vi "Main.vi"() -> ()   [LabVIEW 2018, in "Stream Data.lvlib"]
doc: "This template is based off of the Queued Message Handler design pattern and the Queued Message Handler project template that ships with LabVIEW.\n\nThe main difference is that the queue is private to this module and communication between modules is performed via Broadcast and Request events.\n\nRequest events are wrapped in public API methods and are handled in the Event Handling Loop (EHL) of this VI. Any module can register for Broadcast events sent by this module. The EHL generates messages based on user interface actions.\n\nThe Message Handling Loop (MHL) processes messages generated by the EHL, or by other messages. The messages are string values, so new messages can be added easily to the Message Cases case structure in the MHL. Each message cluster can also provide an optional value for Message Data, which is a variant that can be converted to whatever message-specific data is required.\n_____\nBased on Delacor QMH Project Template 4.2.1.64."
uses:
  Stream Data.lvlib
  <vilib>/Delacor/Delacor QMH/Libraries/Module Admin_class/Delacor_lib_QMH_Module Admin.lvclass
  Private API/Typedefs/CTL_Variable_to_pass.ctl
  Private API/Data.lvclass
  <vilib>/Delacor/Delacor QMH/Libraries/Message Queue_class/Delacor_lib_QMH_Message Queue.lvclass/Delacor_lib_QMH_Message Queue.ctl
  Stop Argument--cluster.ctl
  <vilib>/Delacor/Delacor QMH/Libraries/Module Admin_class/Delacor_lib_QMH_Module Admin.lvclass/Delacor_lib_QMH_Module Admin.ctl
  Send Frame Argument--cluster.ctl
  SubVi's/Controls/CTL_Full_data_frame.ctl
  SubVi's/Controls/CTL_Animal_Coordinates_and_Speed.ctl
  SubVi's/Controls/CTL_Measurements_and_Statistics.ctl
  Open Serial Port Argument--cluster.ctl
  Change Serial Port Argument--cluster.ctl
  Close Serial Port Argument--cluster.ctl
  Update Status Argument--cluster.ctl
  Prepare to Exit Argument--cluster.ctl
  <vilib>/Utility/miscctls.llb/LVPointTypeDef.ctl
  Private API/Data.lvclass/Data.ctl
  <vilib>/Instr/_visa.llb/VISA Open Access Mode.ctl
  <vilib>/Instr/_visa.llb/VISA Set IO Buffer Mask.ctl
  <vilib>/Utility/error.llb/DialogType.ctl
  <vilib>/Delacor/Delacor QMH/Libraries/Message Queue_class/Delacor_lib_QMH_Enqueue Message (Single).vi
  <vilib>/Delacor/Delacor QMH/Libraries/Module Admin_class/Delacor_lib_QMH_Get External Launch.vi
  Private API/Methods/Read Port Opened.vi
  Private API/Methods/Read Serial Port.vi
  Private API/Methods/Write Serial Port.vi
  Private API/Methods/Write Port Opened.vi
  Private API/Methods/Write Status.vi
  <vilib>/Utility/error.llb/Error Cluster From Error Code.vi
  <vilib>/Instr/_visa.llb/VISA Configure Serial Port (Instr).vi
  <vilib>/ErrorRing/Error Ring.xnode
  <vilib>/Delacor/Delacor QMH/Libraries/Message Queue_class/Delacor_lib_QMH_Message Queue.lvclass
  Tracker.lvlib
panel:
  out "Bytes written":u32
  out "Bytes sent":u32
  in  "Line End":u16(ring)=4 items=["Nothing", "Tab", "CR", "LF", "CRLF"]
  in  "Line Start":u16(ring) items=["Nothing", "Tab"]
  in  "Variable 8":T1=enum."Speed, mm/s"
  in  "Variable 7":T1=enum."Zone #"
  in  "Variable 6":T1=enum."Y"
  in  "Variable 5":T1=enum."X"
  in  "Variable 4":T1=enum."alpha"
  in  "Variable 3":T1=enum."phi"
  in  "Variable 2":T1=enum."R"
  in  "Variable 1":T1=enum."timestamp (SW)"
  in  "Mode":bool
  in  "Enable":bool
  in  "Send test frame":bool
  in  "Serial Port":refnum<visa-resource-name>
  in  "Simulate MHL Error":bool
  in  "Simulate EHL Error":bool
  out "error out":errorcluster
  in  "Module Admin":refnum<class "Delacor_lib_QMH_Module Admin.lvclass">
  out "Status":string
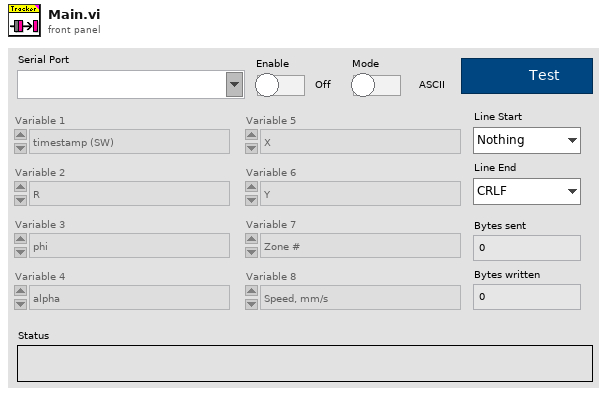
[diagram p1: front panel]
types:
  T1 = typedef "Stream Data.lvlib/CTL_Variable_to_pass.ctl" = enum16{"since ON, ms", "delta time, ms", "timestamp (SW)", "R", "phi", "alpha", "X", "Y", "Zone #", "Run percentage", "Speed, mm/s"}
  T2 = typedef "Stream Data.lvlib/Request Events--cluster.ctl" = cluster{"Stop Module":refnum<user-event>, "Show Panel":refnum<user-event>, "Hide Panel":refnum<user-event>, "Get Module Execution Status":refnum<user-event>, "Show Diagram":refnum<user-event>, "Send Frame":refnum<user-event>, "Open Serial Port":refnum<user-event>, "Change Serial Port":refnum<user-event>, "Close Serial Port":refnum<user-event>, "Update Status":refnum<user-event>, "Prepare to Exit":refnum<user-event>}
  T3 = enum32{"invalid lock state", "Not Locked", "Locked (No Password)", "Password-protected"}
  T4 = typedef "Stream Data.lvlib/Stop Argument--cluster.ctl" = cluster{"Origin":string, "Exit via Stop Module Req?":bool, "Wait for Module to stop?":bool}
  T5 = typedef "Stream Data.lvlib/Send Frame Argument--cluster.ctl" = cluster{"Data in":T6}
  T6 = typedef "Tracker.lvlib/CTL_Full_data_frame.ctl" = cluster{"Times":cluster{"ms since ON":u32, "delta time":u32, "Frame timestamp":timestamp}, "TTLs":cluster{"TTL input":i16, "TTL output":i16}, "Animal coordinates":T7, "Magnets coords raw":cluster{"X1 raw":dbl, "Y1 raw":dbl, "X2 raw":dbl, "Y2 raw":dbl}, "Measurements and statistics":T8}
  T7 = typedef "Tracker.lvlib/CTL_Animal_Coordinates_and_Speed.ctl" = cluster{"R from center":dbl, "phi (mouse angular position in the cage)":dbl, "alpha (mouse rot. angle)":dbl, "X":dbl, "Y":dbl, "theta (from center towards mouse)":dbl, "beta (cage rot. against mouse)":dbl, "w (mouse angle to wall)":dbl, "Speed (filtered)":dbl}
  T8 = typedef "Tracker.lvlib/CTL_Measurements_and_Statistics.ctl" = cluster{"Zone #":i8, "Histogram":dbl[], "Running, perc. of time":dbl, "Run, meters":dbl, "Avg. speed":dbl}
  T9 = typedef "Stream Data.lvlib/Open Serial Port Argument--cluster.ctl" = cluster{"Serial Port":refnum<visa-resource-name>}
  T10 = typedef "Stream Data.lvlib/Change Serial Port Argument--cluster.ctl" = cluster{"Serial Port":refnum<visa-resource-name>}
  T11 = typedef "Stream Data.lvlib/Close Serial Port Argument--cluster.ctl" = cluster{"Serial Port":refnum<visa-resource-name>}
  T12 = typedef "Stream Data.lvlib/Update Status Argument--cluster.ctl" = cluster{"Status":string}
  T13 = typedef "Stream Data.lvlib/Prepare to Exit Argument--cluster.ctl" = cluster{"Boolean":bool}
  T14 = typedef "LVPointTypeDef.ctl" = cluster{"Horizontal":i16, "Vertical":i16}
  T15 = enum32{"Invalid", "Standard", "Closed", "Hidden", "Minimized", "Maximized"}
  T16 = typedef "VISA Set IO Buffer Mask.ctl" = u16
  T17 = typedef "VISA Open Access Mode.ctl" = u32
  T18 = typedef "DialogType.ctl" = u16
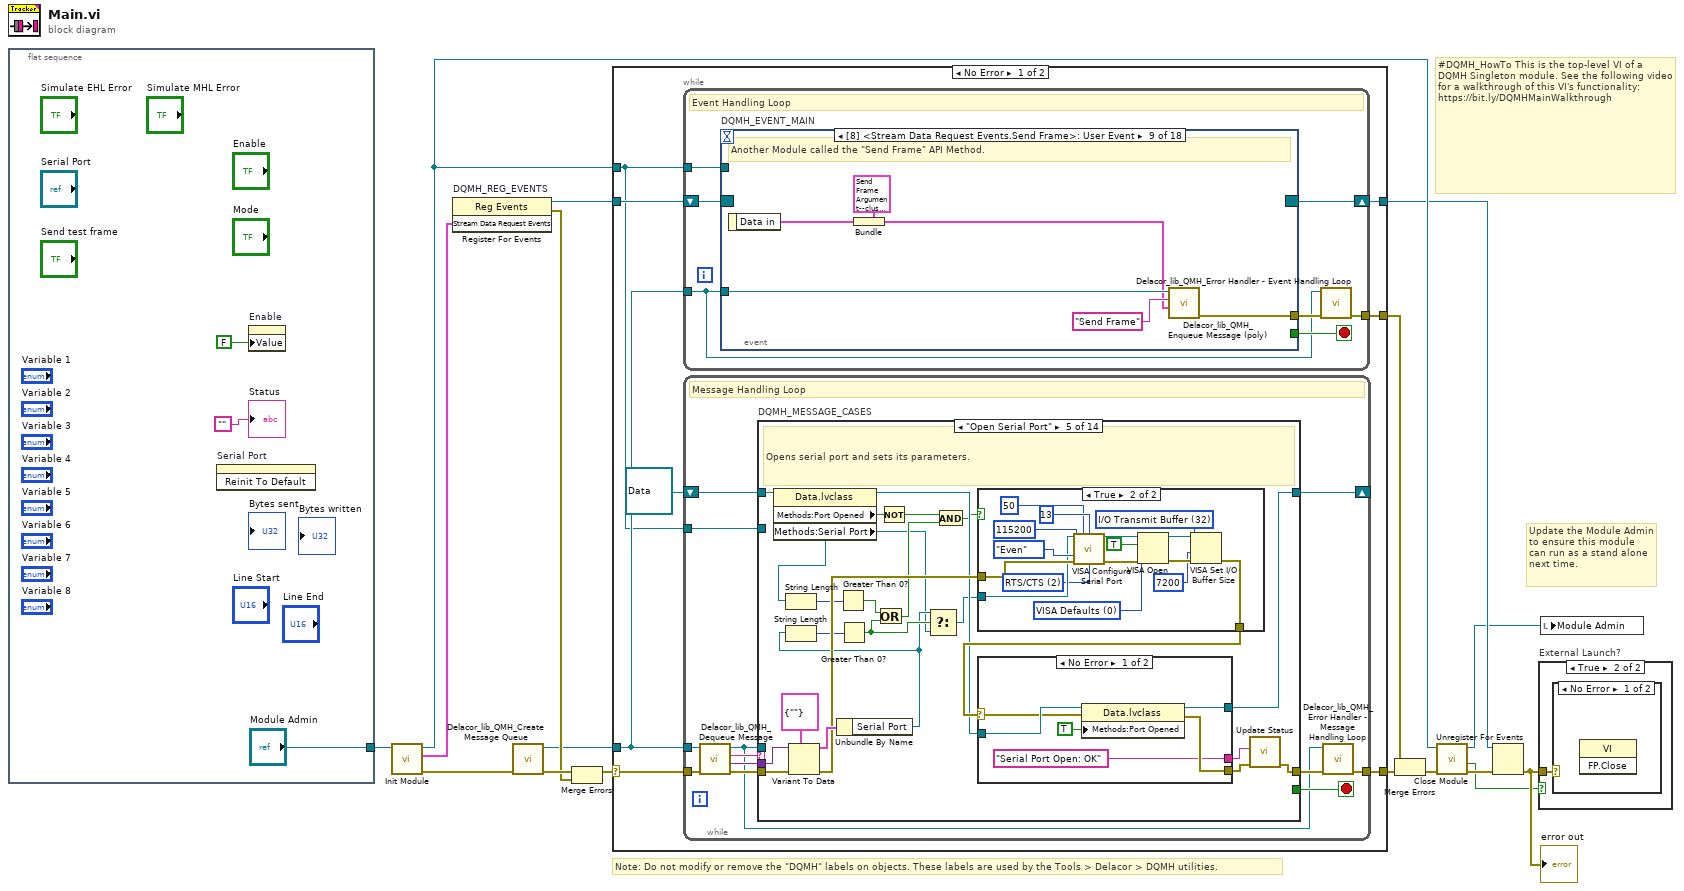
[diagram p0: block diagram]
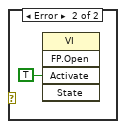
[diagram p3: hidden frame]
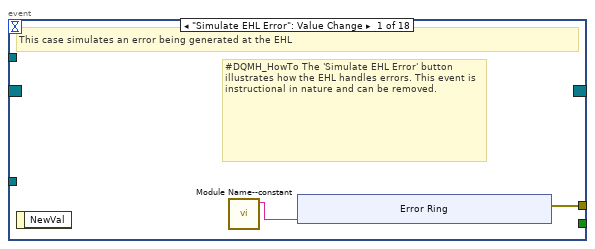
[diagram p4: hidden frame]
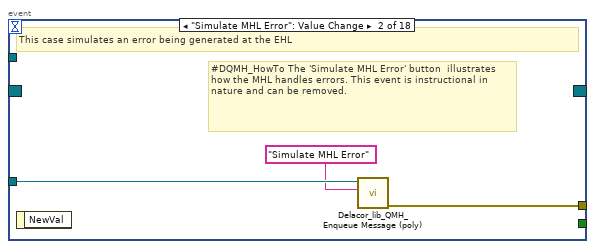
[diagram p5: hidden frame]
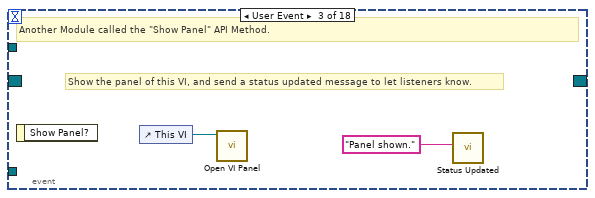
[diagram p6: hidden frame]
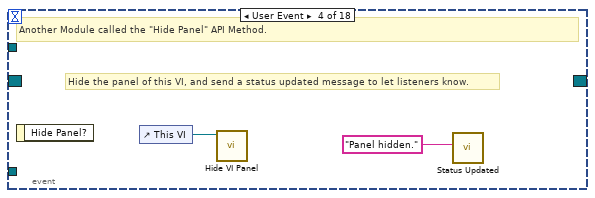
[diagram p7: hidden frame]
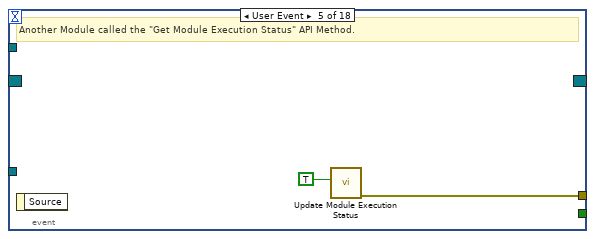
[diagram p8: hidden frame]
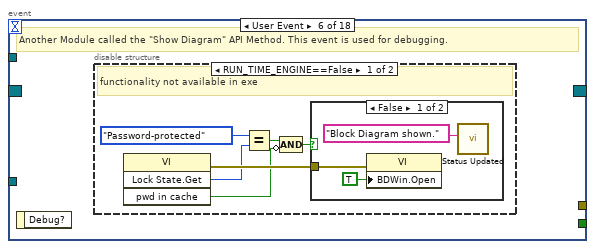
[diagram p9: hidden frame]
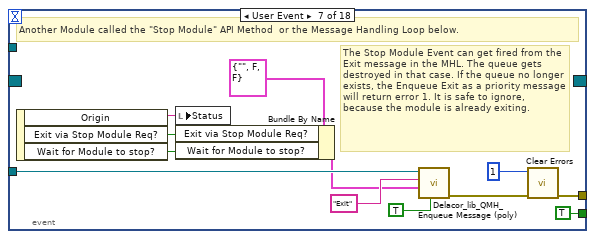
[diagram p12: hidden frame]
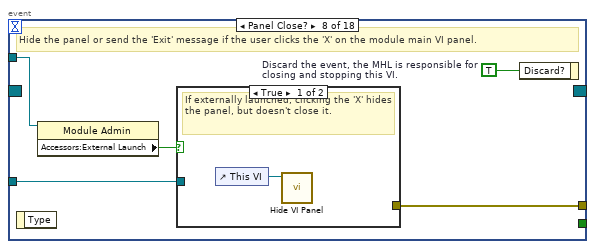
[diagram p13: hidden frame]
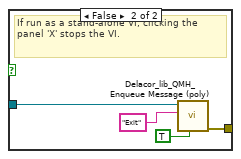
[diagram p14: hidden frame]
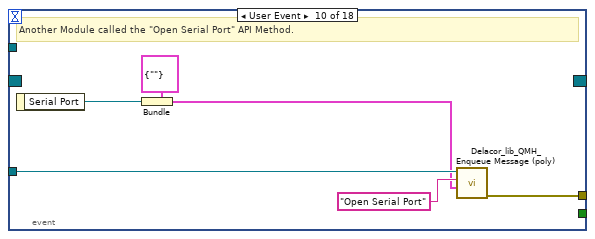
[diagram p15: hidden frame]
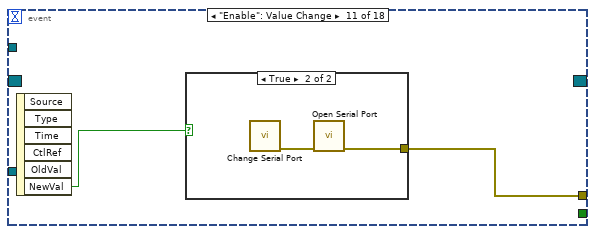
[diagram p16: hidden frame]
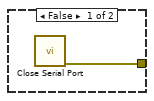
[diagram p17: hidden frame]
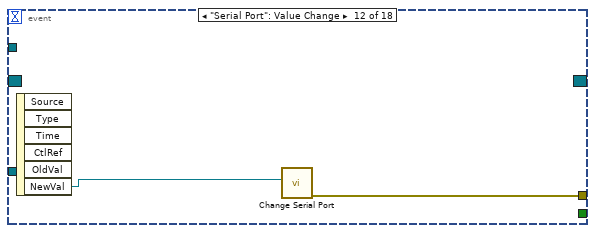
[diagram p18: hidden frame]
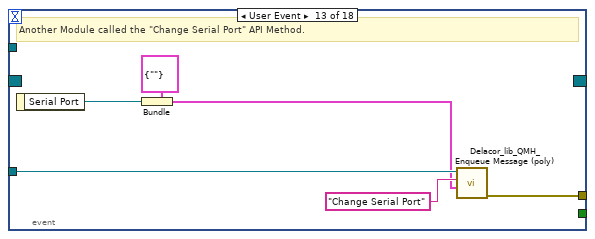
[diagram p19: hidden frame]
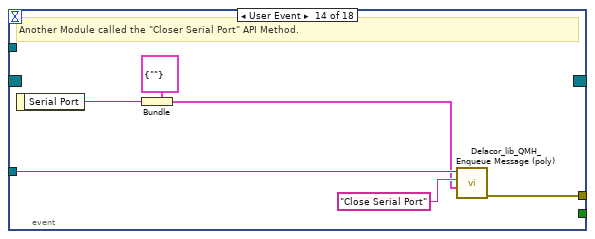
[diagram p20: hidden frame]
diagram:
  # "#DQMH_HowTo This is the top-level VI of a DQMH Singleton module. See the following video for a walkthrough of this VI's functionality: https://bit.ly/DQMHMainWalkthrough"
  # "Note: Do not modify or remove the \"DQMH\" labels on objects. These labels are used by the Tools > Delacor > DQMH utilities."
  # "Update the Module Admin to ensure this module can run as a stand alone next time."
  n1 = flat-sequence {
    tunnel: ["Module Admin"] -> w1
    frame #0 {
      n2 = invoke on="Serial Port" class="VISAName" method="Reinit To Default"() -> ()  [unwired: 3 in, 3 out]
      n3 = property on="Enable" class="Bool (strict)"("Value"=FALSE ("Enable")) -> ()  [unwired: 2 in, 2 out]
      "Status" <- ""
    }
  }
  n4 = call "Init Module.vi"("Singleton Module Admin in"=w1) -> ("error out"=w16:errorcluster, "Stream Data Request Events"=w5:T2, "Singleton Module Admin out"=w8:refnum<class "Delacor_lib_QMH_Module Admin.lvclass">)  [unwired: 8 in]
  n5 = register-events "DQMH_REG_EVENTS"(w5) -> (reference out=w6:refnum<event-registration>, error out=w9:errorcluster)  [unwired: 2 in]
  n6 = call <vilib>:"Delacor_lib_QMH_Create Message Queue.vi"("error in (no error)"=w16) -> ("error out"=w11:errorcluster, "Message Queue"=w4:refnum<class "Delacor_lib_QMH_Message Queue.lvclass">)  [unwired: 9 in]
  n7 = Merge Errors(w11, w9) -> (w10:errorcluster)
  n8 = case shown="No Error" w10 {
    selector: w10 -> [w26 w379]
    tunnel: [w28 w379] -> w17
    tunnel: [w25 w376] -> w7
    tunnel: w6 -> [w24 w376]
    tunnel: w4 -> [w23 _]
    tunnel: [w27 _] -> w14
    tunnel: w8 -> [w22 w372]
    frame No Error {
      n9 = while {
        tunnel: w23 -> [w29]
        shift-right: [w32] -> w25
        shift-left: w24 -> [w33]
        tunnel: [w34] -> w27
        tunnel: w22 -> [w30]
        stop <- w31 stop-if-true
        # "Event Handling Loop"
        n10 = event "DQMH_EVENT_MAIN" shown="[8] <Stream Data Request Events.Send Frame>: User Event" {
          selector: w33 -> [_ _ _ _ _ _ _ _ _ _ _ _ _ _ _ _ _ _]
          dyn-events: [_ _ _ _ _ _ _ _ _ _ _ _ _ _ _ _ _ _] -> w32
          timeout: _ -> [_ _ _ _ _ _ _ _ _ _ _ _ _ _ _ _ _ _]
          tunnel: [_ _ _ _ _ _ TRUE ("Discard?") _ _ _ _ _ _ _ _ _ _ _] -> w31
          tunnel: w29 -> [_ w46 _ _ _ _ w70 w77 w90 w96 _ _ w109 w115 w121 _ _ w131]
          tunnel: [w37 w47 _ _ w53 _ w73 w79 w85 w91 w97 w102 w104 w110 w116 w123 _ w126] -> w35
          tunnel: w30 -> [_ _ _ _ _ _ _ w76 _ _ _ _ _ _ _ _ _ _]
          event "Simulate EHL Error": Value Change {
            # "#DQMH_HowTo The 'Simulate EHL Error' button  illustrates how the EHL handles errors. This event is instructional in nature and can be removed."
            # "This case simulates an error being generated at the EHL"
            n11 = event-data() -> ()  [unwired: 1 in, 1 out]
            n12 = call "Module Name--constant.vi"() -> ("Module Name"=w36:string)  [unwired: 11 in]
            n13 = xnode "Error Ring"("parameter 0"=w36) -> ("error out"=w37:errorcluster)
          }
          event "Simulate MHL Error": Value Change {
            # "#DQMH_HowTo The 'Simulate MHL Error' button  illustrates how the MHL handles errors. This event is instructional in nature and can be removed."
            # "This case simulates an error being generated at the EHL"
            n14 = event-data() -> ()  [unwired: 1 in, 1 out]
            n15 = call-poly <vilib>:"Delacor_lib_QMH_Enqueue Message (poly).vi"("Message"="Simulate MHL Error", "Message Queue in"=w46) -> ("error out"=w47:errorcluster)  [unwired: 8 in, 1 out]
          }
          event User Event {
            # "Show the panel of this VI, and send a status updated message to let listeners know."
            # "Another Module called the \"Show Panel\" API Method."
            n16 = event-data() -> ()  [unwired: 1 in, 1 out]
            n17 = control-ref of="This VI"() -> (w49:refnum<vi>)
            n18 = call "Open VI Panel.vi"("VI"=w49) -> ()  [unwired: 10 in, 1 out]
            n19 = call "Status Updated.vi"("Status"="Panel shown." ("format string")) -> ()  [unwired: 10 in, 1 out]
          }
          event User Event {
            # "Hide the panel of this VI, and send a status updated message to let listeners know."
            # "Another Module called the \"Hide Panel\" API Method."
            n20 = event-data() -> ()  [unwired: 1 in, 1 out]
            n21 = control-ref of="This VI"() -> (w51:refnum<vi>)
            n22 = call "Hide VI Panel.vi"("VI"=w51) -> ()  [unwired: 10 in, 1 out]
            n23 = call "Status Updated.vi"("Status"="Panel hidden." ("format string")) -> ()  [unwired: 10 in, 1 out]
          }
          event User Event {
            # "Another Module called the \"Get Module Execution Status\" API Method."
            n24 = event-data() -> ()  [unwired: 1 in, 1 out]
            n25 = call "Update Module Execution Status.vi"("Running?"=TRUE) -> ("error out"=w53:errorcluster)  [unwired: 10 in]
          }
          event User Event {
            # "Another Module called the \"Show Diagram\" API Method. This event is used for debugging."
            n26 = event-data() -> ()  [unwired: 1 in, 1 out]
            n27 = disable-structure shown="RUN_TIME_ENGINE==False" {
              frame condition #0 (active) {
                # "functionality not available in exe"
                n28 = invoke class="VI" method="Lock State.Get"() -> (error out=w59:errorcluster, "Get Lock State"=w58:T3, "pwd in cache"=w55:bool)  [unwired: 4 in, 1 out]
                n29 = Equal?(x=T3."Password-protected", y=w58) -> (x = y?=w56:bool)
                n30 = Compound Arithmetic op=AND(w56, invert w55) -> (w54:bool)
                n31 = case shown="False" w54 {
                  tunnel: w59 -> [w62 _]
                  frame False {
                    n32 = property class="VI"(error in=w62, "BDWin.Open"=TRUE ("Block Diagram Window:Open")) -> ()  [unwired: 1 in, 2 out]
                    n33 = call "Status Updated.vi"("Status"="Block Diagram shown." ("format string")) -> ()  [unwired: 10 in, 1 out]
                  }
                  frame True {
                    # "Password-protected VI, and the password is not in the cache. Do not show the diagram."
                  }
                }
              }
              frame condition #1 {
              }
            }
          }
          event User Event {
            # "The Stop Module Event can get fired from the Exit message in the MHL. The queue gets destroyed in that case. If the queue no longer exists, the Enqueue Exit as a priority message will return error 1. It is safe to ignore, because the module is already exiting."
            # "Another Module called the \"Stop Module\" API Method  or the Message Handling Loop below."
            n34 = event-data() -> ("Origin"=w69:string, "Exit via Stop Module Req?"=w65:bool, "Wait for Module to stop?"=w64:bool)  [unwired: 1 in]
            n35 = local write "Status"(w69) -> ()
            n36 = Bundle By Name(cluster=T4 {"Origin"="", "Exit via Stop Module Req?"=FALSE, "Wait for Module to stop?"=FALSE} ("Stop Argument"), "Exit via Stop Module Req?"=w65, "Wait for Module to stop?"=w64) -> (w63:T4)
            n37 = call-poly <vilib>:"Delacor_lib_QMH_Enqueue Message (poly).vi"("Priority Message? (F)"=TRUE, "Message Data"=w63, "Message"="Exit", "Message Queue in"=w70) -> ("error out"=w74:errorcluster)  [unwired: 6 in, 1 out]
            n38 = call <vilib>:"Clear Errors.vi"("error in (no error)"=w74, "specific error code to clear (0: all)"=1) -> ("error out"=w73:errorcluster)  [unwired: 4 in, 1 out]
          }
          event Panel Close? {
            w78 = TRUE  # Discard the event, the MHL is responsible for closing and stopping this VI.
            # "Hide the panel or send the 'Exit' message if the user clicks the 'X' on the module main VI panel."
            n39 = event-data() -> ()  [unwired: 1 in, 1 out]
            n40 = property class="Module Admin"(reference=w76) -> ("Accessors:External Launch"=w75:bool)  [unwired: 1 in, 2 out]
            n41 = case shown="True" w75 {
              tunnel: w77 -> [_ w83]
              tunnel: [_ w84] -> w79
              frame True {
                # "If externally launched, clicking the 'X' hides the panel, but doesn't close it."
                n42 = control-ref of="This VI"() -> (w80:refnum<vi>)
                n43 = call "Hide VI Panel.vi"("VI"=w80) -> ()  [unwired: 10 in, 1 out]
              }
              frame False {
                # "If run as a stand-alone VI, clicking the panel 'X' stops the VI."
                n44 = call-poly <vilib>:"Delacor_lib_QMH_Enqueue Message (poly).vi"("Priority Message? (F)"=TRUE, "Message"="Exit", "Message Queue in"=w83) -> ("error out"=w84:errorcluster)  [unwired: 7 in, 1 out]
              }
            }
            n45 = event-data("Discard?"=w78) -> ()  [unwired: 1 in, 1 out]
          }
          event User Event {
            # "Another Module called the \"Send Frame\" API Method."
            n46 = event-data() -> ("Data in"=w86:T6)  [unwired: 1 in]
            n47 = Bundle(cluster=T5 {"Data in"={"Times"={"ms since ON"=0, "delta time"=0, "Frame timestamp"=timestamp(0 s since 1904-01-01)}, "TTLs"={"TTL input"=0, "TTL output"=0}, "Animal coordinates"={"R from center"=0.0, "phi (mouse angular position in the cage)"=0.0, "alpha (mouse rot. angle)"=0.0, "X"=0.0, "Y"=0.0, "theta (from center towards mouse)"=0.0, "beta (cage rot. against mouse)"=0.0, "w (mouse angle to wall)"=0.0, "Speed (filtered)"=0.0}, "Magnets coords raw"={"X1 raw"=0.0, "Y1 raw"=0.0, "X2 raw"=0.0, "Y2 raw"=0.0}, "Measurements and statistics"={"Zone #"=0, "Histogram"=[], "Running, perc. of time"=0.0, "Run, meters"=0.0, "Avg. speed"=0.0}}} ("Send Frame Argument"), "Data in"=w86) -> (w87:T5)
            n48 = call-poly <vilib>:"Delacor_lib_QMH_Enqueue Message (poly).vi"("Message Data"=w87, "Message"="Send Frame", "Message Queue in"=w90) -> ("error out"=w85:errorcluster)  [unwired: 7 in, 1 out]
          }
          event User Event {
            # "Another Module called the \"Open Serial Port\" API Method."
            n49 = event-data() -> ("Serial Port"=w92:refnum<visa-resource-name>)  [unwired: 1 in]
            n50 = Bundle(cluster=T9 {"Serial Port"=""} ("Open Serial Port Argument"), "Serial Port"=w92) -> (w93:T9)
            n51 = call-poly <vilib>:"Delacor_lib_QMH_Enqueue Message (poly).vi"("Message Data"=w93, "Message"="Open Serial Port", "Message Queue in"=w96) -> ("error out"=w91:errorcluster)  [unwired: 7 in, 1 out]
          }
          event "Enable": Value Change {
            n52 = event-data() -> ("NewVal"=w98:bool)  [unwired: 1 in, 5 out]
            n53 = case shown="True" w98 {
              tunnel: [w99 w101] -> w97
              frame False {
                n54 = call "Close Serial Port.vi"() -> ("error out"=w99:errorcluster)  [unwired: 11 in]
              }
              frame True {
                n55 = call "Change Serial Port.vi"() -> ("error out"=w100:errorcluster)  [unwired: 11 in]
                n56 = call "Open Serial Port.vi"("error in (no error)"=w100) -> ("error out"=w101:errorcluster)  [unwired: 10 in]
              }
            }
          }
          event "Serial Port": Value Change {
            n57 = event-data() -> ("NewVal"=w103:refnum<visa-resource-name>)  [unwired: 1 in, 5 out]
            n58 = call "Change Serial Port.vi"("Serial Port"=w103) -> ("error out"=w102:errorcluster)  [unwired: 10 in]
          }
          event User Event {
            # "Another Module called the \"Change Serial Port\" API Method."
            n59 = event-data() -> ("Serial Port"=w105:refnum<visa-resource-name>)  [unwired: 1 in]
            n60 = Bundle(cluster=T10 {"Serial Port"=""} ("Change Serial Port Argument"), "Serial Port"=w105) -> (w106:T10)
            n61 = call-poly <vilib>:"Delacor_lib_QMH_Enqueue Message (poly).vi"("Message Data"=w106, "Message"="Change Serial Port", "Message Queue in"=w109) -> ("error out"=w104:errorcluster)  [unwired: 7 in, 1 out]
          }
          event User Event {
            # "Another Module called the \"Closer Serial Port\" API Method."
            n62 = event-data() -> ("Serial Port"=w111:refnum<visa-resource-name>)  [unwired: 1 in]
            n63 = Bundle(cluster=T11 {"Serial Port"=""} ("Closer Serial Port Argument"), "Serial Port"=w111) -> (w112:T11)
            n64 = call-poly <vilib>:"Delacor_lib_QMH_Enqueue Message (poly).vi"("Message Data"=w112, "Message"="Close Serial Port", "Message Queue in"=w115) -> ("error out"=w110:errorcluster)  [unwired: 7 in, 1 out]
          }
          event User Event {
            # "Another Module called the \"Update Status\" API Method."
            n65 = event-data() -> ("Status"=w117:string)  [unwired: 1 in]
            n66 = Bundle(cluster=T12 {"Status"=""} ("Update Status Argument"), "Status"=w117) -> (w118:T12)
            n67 = call-poly <vilib>:"Delacor_lib_QMH_Enqueue Message (poly).vi"("Message Data"=w118, "Message"="Update Status", "Message Queue in"=w121) -> ("error out"=w116:errorcluster)  [unwired: 7 in, 1 out]
          }
          event "Send test frame": Value Change {
            n68 = event-data() -> ("OldVal"=w125:bool)  [unwired: 1 in, 5 out]
            n69 = property on="Send test frame" class="Bool (strict)"("Value"=w125) -> ()  [unwired: 2 in, 2 out]
            n70 = call "SD_Gen_Random_Frame.vi"() -> ("error out"=w124:errorcluster, "Generated data"=w122:T6)  [unwired: 10 in]
            n71 = call "Send Frame.vi"("error in (no error)"=w124, "Data in"=w122) -> ("error out"=w123:errorcluster)  [unwired: 9 in]
          }
          event Value Change {
            n72 = event-data() -> ()  [unwired: 1 in, 6 out]
          }
          event User Event {
            # "Another Module called the \"Prepare to Exit\" API Method."
            n73 = event-data() -> ("Boolean"=w127:bool)  [unwired: 1 in]
            n74 = Bundle(cluster=T13 {"Boolean"=FALSE} ("Prepare to Exit Argument"), "Boolean"=w127) -> (w128:T13)
            n75 = call-poly <vilib>:"Delacor_lib_QMH_Enqueue Message (poly).vi"("Message Data"=w128, "Message"="Prepare to Exit", "Message Queue in"=w131) -> ("error out"=w126:errorcluster)  [unwired: 7 in, 1 out]
          }
        }
        n76 = call-dynamic "Delacor_lib_QMH_Error Handler - Event Handling Loop.vi"("error in (no error)"=w35, "Message Queue in"=w29) -> ("dup error in"=w34:errorcluster)  [unwired: 8 in, 1 out]
      }
      n77 = while {
        tunnel: w23 -> [w134]
        shift-right: [w138] -> _
        shift-left: refnum<class "Data.lvclass"> refnum ("Stream Data.lvlib:Data.lvclass") -> [w139]
        tunnel: w26 -> [w142]
        tunnel: [w140] -> w28
        tunnel: w22 -> [w132]
        stop <- w137 stop-if-true
        # "Message Handling Loop"
        n78 = call-dynamic "Delacor_lib_QMH_Dequeue Message.vi"("error in (no error)"=w142, "Message Queue in"=w134) -> ("error out"=w141:errorcluster, "Message Data"=w135:variant, "Message"=w136:string, "Message Queue out"=w133:refnum<class "Delacor_lib_QMH_Message Queue.lvclass">)  [unwired: 6 in]
        n79 = case "DQMH_MESSAGE_CASES" shown="\"Open Serial Port\"" w136 {
          selector: w136 -> [_ _ _ _ _ _ _ _ _ _ _ _ _ w359]
          tunnel: w133 -> [_ _ _ _ _ _ _ _ _ _ _ w325 w351 _]
          tunnel: w141 -> [w160 w164 w173 w201 w224 w268 w295 w305 w308 w310 w315 w332 w357 w361]
          tunnel: [w158 w164 w166 w189 w203 w255 w293 w300 w307 w310 w314 w328 w354 w362] -> w143
          tunnel: w139 -> [w145 w163 w170 w200 w223 w267 w294 w304 w306 w309 w312 w327 w350 w360]
          tunnel: [w145 w163 w170 w196 w215 w257 w289 w304 w306 w309 w312 w327 w350 w360] -> w138
          tunnel: [_ _ _ _ _ _ _ _ _ _ _ _ w349 _] -> w137
          tunnel: w135 -> [_ _ w172 w199 w222 w266 w292 w303 _ _ _ w326 w348 _]
          tunnel: w132 -> [w150 _ _ _ _ _ _ _ _ _ _ w324 w343 _]
          frame "Initialize" {
            # "Initialize - Any operation that needs to be done before the module can receive messages. Synchronize Caller Events.vi will inform Start Module.vi that the module has launched and is ready to receive messages. Module Did Init.vi will broadcast that the module initialized."
            n80 = call "Synchronize Caller Events.vi"("error in (no error)"=w160, "Singleton Module Admin in"=w150) -> ("error out"=w159:errorcluster, "Singleton Module Admin out"=w147:refnum<class "Delacor_lib_QMH_Module Admin.lvclass">)  [unwired: 8 in]
            n81 = property class="Module Admin"(reference=w147) -> ("Accessors:External Launch"=w154:bool)  [unwired: 1 in, 2 out]
            n82 = Select(t=T15."Hidden" ("State"), s=w154, f=T15."Standard" ("State")) -> (s? t:f=w151:T15)
            n83 = call "Module Name--constant.vi"() -> ("Module Name"=w157:string)  [unwired: 11 in]
            n84 = property class="VI"("Front Panel.Title"=w157) -> (reference out=w156:refnum<vi>, error out=w162:errorcluster)  [unwired: 2 in]
            n85 = call "Update Status.vi"("Status"="Initial Message" ("Initial Message")) -> ()  [unwired: 10 in, 1 out]
            n86 = call "Module Name--constant.vi"() -> ("Module Name"=w148:string)  [unwired: 11 in]
            n87 = invoke class="VI" method="FP.Open"(reference=w156, error in=w162, "State"=w151) -> (reference out=w155:refnum<vi>, error out=w161:errorcluster)  [unwired: 2 in, 3 out]
            n88 = call "Module Did Init.vi"("error in (no error)"=w159, "Initialized?"=TRUE, "Origin"=w148) -> ("error out"=w158:errorcluster)  [unwired: 8 in]
            n89 = invoke class="VI" method="FP.Center"(reference=w155, error in=w161) -> ()  [unwired: 1 in, 3 out]
            n90 = property on="Pane" class="Pane"("Origin"=T14 {"Horizontal"=0, "Vertical"=0}) -> ()  [unwired: 2 in, 2 out]
          }
          frame "--- Module Specific ---" {
            # "Separator -- The following cases handle messages specific to this Module."
          }
          frame "Send Frame" {
            # "Requests to send a single data frame."
            n91 = property class="Data.lvclass"(reference=w170) -> ("Methods:Port Opened"=w169:bool, "Methods:Serial Port"=w165:refnum<visa-resource-name>)  [unwired: 1 in, 2 out]
            n92 = Variant To Data(error in=w173, type=T5 {"Data in"={"Times"={"ms since ON"=0, "delta time"=0, "Frame timestamp"=timestamp(0 s since 1904-01-01)}, "TTLs"={"TTL input"=0, "TTL output"=0}, "Animal coordinates"={"R from center"=0.0, "phi (mouse angular position in the cage)"=0.0, "alpha (mouse rot. angle)"=0.0, "X"=0.0, "Y"=0.0, "theta (from center towards mouse)"=0.0, "beta (cage rot. against mouse)"=0.0, "w (mouse angle to wall)"=0.0, "Speed (filtered)"=0.0}, "Magnets coords raw"={"X1 raw"=0.0, "Y1 raw"=0.0, "X2 raw"=0.0, "Y2 raw"=0.0}, "Measurements and statistics"={"Zone #"=0, "Histogram"=[], "Running, perc. of time"=0.0, "Run, meters"=0.0, "Avg. speed"=0.0}}} ("Send Frame Argument"), Variant=w172) -> (data=w167:T5, error out=w168:errorcluster)
            n93 = case shown="True" w169 {
              tunnel: w168 -> [w174 w184]
              tunnel: w167 -> [_ w183]
              tunnel: [w174 w181] -> w166
              tunnel: w165 -> [_ w180]
              frame False {
              }
              frame True {
                n94 = local read "Line Start"() -> (w178:u16)
                n95 = local read "Mode"() -> (w185:bool)
                n96 = local read "Line End"() -> (w177:u16)
                n97 = call "SD_Construct_data_string.vi"("Line End"=w177, "Line Start"=w178, "error in (no error)"=w184, "Mode"=w185, "Send Frame Argument"=w183) -> ("error out"=w182:errorcluster, "Total bytes"=w176:i32, "Data string"=w179:string)  [unwired: 4 in]
                n98 = local write "Bytes sent"(w176) -> ()
                n99 = VISA Write(VISA resource name=w180, write buffer=w179, error in (no error)=w182) -> (return count=w175:u32, error out=w181:errorcluster)  [unwired: 1 out]
                n100 = local write "Bytes written"(w175) -> ()
              }
            }
          }
          frame "Change Serial Port" {
            # "Changes current serial port information in the class data."
            n101 = Variant To Data(error in=w201, type=T10 {"Serial Port"=""} ("Change Serial Port Argument"), Variant=w199) -> (data=w197:T10, error out=w195:errorcluster)
            n102 = Unbundle By Name(w197) -> ("Serial Port"=w191:refnum<visa-resource-name>)
            n103 = String Length(string=w191) -> (length=w194:i32)
            n104 = local read "Serial Port"() -> (w192:refnum<visa-resource-name>)
            n105 = Greater Than 0?(x=w194) -> (x > 0?=w193:bool)
            n106 = Select(t=w191, s=w193, f=w192) -> (s? t:f=w186:refnum<visa-resource-name>)
            n107 = property class="Data.lvclass"(reference=w200, error in=w195, "Methods:Serial Port"=w186) -> (reference out=w196:refnum<class "Data.lvclass">, error out=w190:errorcluster)
            n108 = Concatenate Strings("Serial port class data changed to: " ("Status"), w186) -> (w187:string)
            n109 = call "Update Status.vi"("error in (no error)"=w190, "Status"=w187) -> ("error out"=w189:errorcluster)  [unwired: 9 in]
          }
          frame "Open Serial Port" {
            # "Opens serial port and sets its parameters."
            n110 = property class="Data.lvclass"(reference=w223) -> (reference out=w216:refnum<class "Data.lvclass">, "Methods:Port Opened"=w219:bool, "Methods:Serial Port"=w206:refnum<visa-resource-name>)  [unwired: 1 in, 1 out]
            n111 = String Length(string=w206) -> (length=w212:i32)
            n112 = Variant To Data(error in=w224, type=T9 {"Serial Port"=""} ("Open Serial Port Argument"), Variant=w222) -> (data=w220:T9, error out=w218:errorcluster)
            n113 = Unbundle By Name(w220) -> ("Serial Port"=w207:refnum<visa-resource-name>)
            n114 = String Length(string=w207) -> (length=w211:i32)
            n115 = Greater Than 0?(x=w212) -> (x > 0?=w210:bool)
            n116 = Greater Than 0?(x=w211) -> (x > 0?=w208:bool)
            n117 = Or(x=w210, y=w208) -> (x .or. y?=w209:bool)
            n118 = Not(x=w219) -> (.not. x?=w213:bool)
            n119 = Select(t=w207, s=w208, f=w206) -> (s? t:f=w205:refnum<visa-resource-name>)
            n120 = And(x=w213, y=w209) -> (x .and. y?=w214:bool)
            n121 = case shown="True" w214 {
              tunnel: w218 -> [w237 w253]
              tunnel: [w237 w245] -> w217
              tunnel: w205 -> [_ w241]
              frame False {
              }
              frame True {
                w239 = u16 2 items=["None", "XON/XOFF", "RTS/CTS", "XON/XOFF & RTS/CTS", "DTR/DSR", "XON/XOFF & DTR/DSR"] ("flow control (0:none)")
                w243 = T16 32 items=["I/O Receive Buffer"=16, "I/O Transmit Buffer"=32, "I/O Receive and Transmit Buffer"=48] ("Mask")
                w247 = T17 0 items=["VISA Defaults"=0, "Exclusive Lock"=1, "Load Configured Settings"=4] ("Access Mode")
                n122 = call-poly "VISA Configure Serial Port"("VISA resource name"=w241, "timeout (10sec)"=u32 50, "termination char\n(0xA = '\\n' = LF)"=u8 13 ("termination char\n(0xA = '\\n' = LF)"), "baud rate (9600)"=u32 115200, "parity (0:none)"=enum16{"None", "Odd", "Even", "Mark", "Space"}."Even", "error in (no error)"=w253, "flow control (0:none)"=w239) -> ("VISA resource name out"=w249:refnum<visa-resource-name>, "error out"=w248:errorcluster)  [unwired: 7 in]
                n123 = VISA Open(duplicate session (F)=TRUE, access mode=w247, error in (no error)=w248, VISA resource name=w249) -> (VISA resource name=w244:refnum<visa-resource-name>, error out=w246:errorcluster)  [unwired: 1 in]
                n124 = VISA Set I/O Buffer Size(VISA resource name=w244, mask (16)=w243, size (4096)=u32 7200, error in (no error)=w246) -> (error out=w245:errorcluster)  [unwired: 1 out]
              }
            }
            n125 = case shown="No Error" w217 {
              selector: w217 -> [w229 w235]
              tunnel: w216 -> [w230 w236]
              tunnel: [w228 w234] -> w215
              tunnel: [w227 w233] -> w204
              tunnel: ["Serial Port Open: OK" ("Status") "Serial Port Open: FAILED" ("Status")] -> w202
              frame No Error {
                n126 = property class="Data.lvclass"(reference=w230, error in=w229, "Methods:Port Opened"=TRUE ("Port Opened")) -> (reference out=w228:refnum<class "Data.lvclass">, error out=w227:errorcluster)
              }
              frame Error {
                n127 = property class="Data.lvclass"(reference=w236, error in=w235, "Methods:Port Opened"=FALSE ("Port Opened")) -> (reference out=w234:refnum<class "Data.lvclass">, error out=w233:errorcluster)
              }
            }
            n128 = call "Update Status.vi"("error in (no error)"=w204, "Status"=w202) -> ("error out"=w203:errorcluster)  [unwired: 9 in]
          }
          frame "Close Serial Port" {
            # "Closes the previously opened serial port."
            n129 = property class="Data.lvclass"(reference=w267) -> (reference out=w258:refnum<class "Data.lvclass">, "Methods:Port Opened"=w263:bool, "Methods:Serial Port"=w262:refnum<visa-resource-name>)  [unwired: 1 in, 1 out]
            n130 = Variant To Data(error in=w268, type=T11 {"Serial Port"=""} ("Closer Serial Port Argument"), Variant=w266) -> (data=w264:T11, error out=w260:errorcluster)
            n131 = Unbundle By Name(w264) -> ("Serial Port"=w261:refnum<visa-resource-name>)
            n132 = case shown="True" w263 {
              tunnel: w261 -> [_ w279]
              tunnel: w262 -> [_ w285]
              tunnel: w260 -> [w278 w281]
              tunnel: [w278 w280] -> w259
              frame False {
              }
              frame True {
                n133 = String Length(string=w279) -> (length=w287:i32)
                n134 = Greater Than 0?(x=w287) -> (x > 0?=w286:bool)
                n135 = Select(t=w279, s=w286, f=w285) -> (s? t:f=w284:refnum<visa-resource-name>)
                n136 = VISA Flush I/O Buffer(VISA resource name=w284, error in (no error)=w281) -> (VISA resource name out=w283:refnum<visa-resource-name>, error out=w282:errorcluster)  [unwired: 1 in]
                n137 = VISA Close(VISA resource name=w283, error in (no error)=w282) -> (error out=w280:errorcluster)
              }
            }
            n138 = case shown="No Error" w259 {
              selector: w259 -> [w273 w276]
              tunnel: w258 -> [w274 w277]
              tunnel: [w272 w277] -> w257
              tunnel: [w271 w276] -> w256
              tunnel: ["Serial Port Close: OK" ("Status") "Serial Port Close: FAILED" ("Status")] -> w254
              frame No Error {
                n139 = property class="Data.lvclass"(reference=w274, error in=w273, "Methods:Port Opened"=FALSE ("Port Opened")) -> (reference out=w272:refnum<class "Data.lvclass">, error out=w271:errorcluster)
              }
              frame Error {
              }
            }
            n140 = call "Update Status.vi"("error in (no error)"=w256, "Status"=w254) -> ("error out"=w255:errorcluster)  [unwired: 9 in]
          }
          frame "Update Status" {
            # "Updates status with a given string."
            n141 = Variant To Data(error in=w295, type=T12 {"Status"=""} ("Update Status Argument"), Variant=w292) -> (data=w290:T12, error out=w293:errorcluster)
            n142 = Unbundle By Name(w290) -> ("Status"=w288:string)
            n143 = property class="Data.lvclass"(reference=w294, "Methods:Status"=w288) -> (reference out=w289:refnum<class "Data.lvclass">)  [unwired: 1 in, 1 out]
            n144 = local write "Status"(w288) -> ()
          }
          frame "Prepare to Exit" {
            # "Initiates Exit sequence."
            n145 = Variant To Data(error in=w305, type=T13 {"Boolean"=FALSE} ("Prepare to Exit Argument"), Variant=w303) -> (error out=w301:errorcluster)  [unwired: 1 out]
            n146 = call "Close Serial Port.vi"("error in (no error)"=w301) -> ("error out"=w299:errorcluster)  [unwired: 10 in]
            n147 = call "Update Status.vi"("error in (no error)"=w299, "Status"="Stream data exit sequence initiated.") -> ("error out"=w298:errorcluster)  [unwired: 9 in]
            n148 = call "Stop Module.vi"("Timeout to Wait for Stop (s) (-1: no timeout)"=5.0, "error in (no error)"=w298) -> ("error out"=w300:errorcluster)  [unwired: 9 in]
          }
          frame "---Copy This Frame---" {
            # "Duplicate this frame when creating new messages.  Change this comment in the duplicated frame to describe this message."
            n149 = Merge Errors(w308) -> (w307:errorcluster)
          }
          frame "--- Exit and Error Handling---" {
            # "Separator - The following cases handle errors and exit messages."
          }
          frame "Simulate MHL Error" {
            # "#DQMH_HowTo The 'Simulate MHL Error' button  illustrates how the MHL handles errors. This event is instructional in nature and can be removed."
            # "Simulate an error occurring at the MHL"
            n150 = call "Module Name--constant.vi"() -> ("Module Name"=w311:string)  [unwired: 11 in]
            n151 = xnode "Error Ring"("parameter 0"=w311) -> ("error out"=w313:errorcluster)
            n152 = Merge Errors(w315, w313) -> (w314:errorcluster)
          }
          frame "Error" {
            # "#CodeRecommended - If you ever change the name of this \"Error\" message, you'll need to update the name in the Check Loop Error.vi as well."
            # "#CodeRecommended - If the module is running in standalone mode (External Launch = FALSE), this code will pop up an error dialog and call the 'Exit' message if an error occurs. Add more fine-grained error handling here."
            # "Error - Check the error message data and respond accordingly. This message is sent by the \"Error Handler\" VIs at the end of each loop in this application."
            n153 = property class="Module Admin"(reference=w324) -> ("Accessors:External Launch"=w323:bool)  [unwired: 1 in, 2 out]
            n154 = Variant To Data(error in=w332, type=errorcluster {"status"=FALSE, "code"=0, "source"=""} ("error constant"), Variant=w326) -> (data=w333:errorcluster, error out=w330:errorcluster)
            n155 = call "Error Reported.vi"("Error"=w333) -> ()  [unwired: 10 in, 1 out]
            n156 = case shown="False" w323 {
              tunnel: [w336 w338] -> w329
              tunnel: w325 -> [_ _]
              tunnel: w333 -> [w337 w342]
              frame False {
                n157 = call <vilib>:"Simple Error Handler.vi"("error in (no error)"=w337) -> ("error out"=w335:errorcluster, "message"=w334:string)  [unwired: 4 in, 3 out]
                n158 = call "Update Status.vi"("Status"=w334) -> ()  [unwired: 10 in, 1 out]
                n159 = call <vilib>:"Clear Errors.vi"("error in (no error)"=w335) -> ("error out"=w336:errorcluster)  [unwired: 5 in, 1 out]
              }
              frame True {
                w341 = T18 0 items=["no dialog", "OK message", "continue or stop message", "OK message + warnings", "continue/stop + warnings"] ("type of dialog (OK msg:1)")
                n160 = call <vilib>:"Simple Error Handler.vi"("type of dialog (OK msg:1)"=w341, "error in (no error)"=w342) -> ("error out"=w339:errorcluster, "message"=w340:string)  [unwired: 3 in, 3 out]
                n161 = call "Update Status.vi"("Status"=w340) -> ()  [unwired: 10 in, 1 out]
                n162 = call <vilib>:"Clear Errors.vi"("error in (no error)"=w339) -> ("error out"=w338:errorcluster)  [unwired: 5 in, 1 out]
              }
            }
            n163 = Merge Errors(w330, w329) -> (w328:errorcluster)
            n164 = local write "error out"(w328) -> ()
          }
          frame "Exit" {
            w347 = 91  # 91: not all Exit messages will have an argument
            w349 = TRUE  # Stop the VI
            # "Release the message queue reference"
            # "#CodeNeeded - Add any required cleanup code here"
            # "Exit - Exit the application."
            n165 = Variant To Data(error in=w357, type=T4 {"Origin"="", "Exit via Stop Module Req?"=FALSE, "Wait for Module to stop?"=FALSE} ("Stop Argument"), Variant=w348) -> (data=w345:T4, error out=w353:errorcluster)
            n166 = call <vilib>:"Clear Errors.vi"("error in (no error)"=w353, "specific error code to clear (0: all)"=w347) -> ("error out"=w356:errorcluster)  [unwired: 4 in, 1 out]
            n167 = control-ref of="This VI"() -> (w344:refnum<vi>)
            n168 = call-dynamic "Delacor_lib_QMH_Release Message Queue.vi"("error in (no error)"=w356, "Message Queue"=w351) -> ("error out"=w355:errorcluster)  [unwired: 9 in]
            n169 = call "Handle Exit.vi"("Stop Argument"=w345, "Admin in"=w343, "VI reference"=w344) -> ("error out"=w352:errorcluster)  [unwired: 7 in, 1 out]
            n170 = Merge Errors(w355, w352) -> (w354:errorcluster)
          }
          frame Default {
            # "'Default' case only runs if there is a message that isn't defined in any of the other cases.  Output a programming error."
            n171 = call "Module Name--constant.vi"() -> ("Module Name"=w358:string)  [unwired: 11 in]
            n172 = xnode "Error Ring"("parameter 0"=w359, "parameter 1"=w358) -> ("error out"=w363:errorcluster)
            n173 = Merge Errors(w361, w363) -> (w362:errorcluster)
          }
        }
        n174 = call-dynamic "Delacor_lib_QMH_Error Handler - Message Handling Loop.vi"("error in (no error)"=w143, "Message Queue in"=w133) -> ("dup error in"=w140:errorcluster)  [unwired: 8 in, 1 out]
      }
    }
    frame Error {
      # "Synchronize Caller Events.vi will inform Start Module.vi that the module has launched and will let the code calling Start Module.vi register for broadcasts and would permit the caller receive the broadcast that an error occurred at launch time."
      n175 = call "Synchronize Caller Events.vi"("Singleton Module Admin in"=w372) -> ("error out"=w377:errorcluster)  [unwired: 9 in, 1 out]
      n176 = call "Module Name--constant.vi"() -> ("Module Name"=w375:string)  [unwired: 11 in]
      n177 = Format Into String(format string="An error occurred during initialization. %s is no longer running.", w375) -> (resulting string=w373:string)  [unwired: 2 in, 1 out]
      n178 = Merge Errors(w379, w377) -> (w378:errorcluster)
      n179 = call "Error Reported.vi"("Additional Information"=w373, "Error"=w378) -> ()  [unwired: 9 in, 1 out]
    }
  }
  n180 = Merge Errors(w14, w17) -> (w13:errorcluster)
  n181 = call "Close Module.vi"("error in (no error)"=w13, "Module Admin in"=w8) -> ("error out"=w15:errorcluster, "External Launch"=w2:bool, "Module Admin out"=w3:refnum<class "Delacor_lib_QMH_Module Admin.lvclass">)  [unwired: 7 in]
  n182 = Unregister For Events(event registration refnum=w7, error in=w15) -> (error out=w12:errorcluster)
  "error out" <- w12
  n183 = case "External Launch?" shown="True" w2 {
    tunnel: w12 -> [_ w380]
    frame False {
    }
    frame True {
      n184 = case shown="No Error" w380 {
        frame No Error {
          n185 = invoke class="VI" method="FP.Close"() -> ()  [unwired: 3 in, 3 out]
        }
        frame Error {
          n186 = invoke class="VI" method="FP.Open"("Activate"=TRUE ("Activate?")) -> ()  [unwired: 4 in, 5 out]
        }
      }
    }
  }
  n187 = local write "Module Admin"(w3) -> ()
